vi "Pack Message Identifier.vi"(10 "message identifiers":cluster{"Port":u8, "Label":u8, "SDI":u8}) -> (2 "packed message identifier":u32)   [LabVIEW 2020]
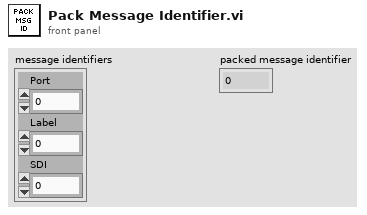
[diagram p1: front panel]
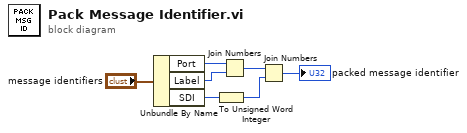
[diagram p0: block diagram]
diagram:
  n1 = Unbundle By Name("message identifiers") -> ("Port"=w6:u8, "Label"=w5:u8, "SDI"=w2:u8)
  n2 = To Unsigned Word Integer(number=w2) -> (unsigned 16bit integer=w1:u16)
  n3 = Join Numbers(hi=w6, lo=w5) -> ((hi.lo)=w4:u16)
  n4 = Join Numbers(hi=w4, lo=w1) -> ((hi.lo)=→"packed message identifier":u32)
